vi "Dec.vi"(8 "error in (no error)":errorcluster) -> (0 "error out":errorcluster, 3 "function return":dbl)   [LabVIEW 2014, in "MASTTCSGET.lvlib"]
doc: "gives teliscope declination\n\n\n\n\n__declspec (dllexport) float Dec();"
uses:
  MASTTCSGET.lvlib
  MASTTCSGET.dll
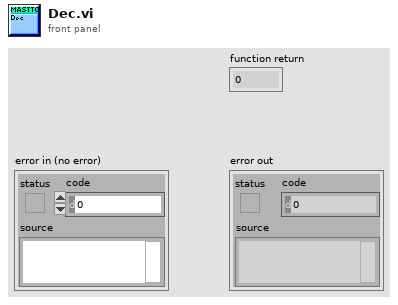
[diagram p1: front panel]
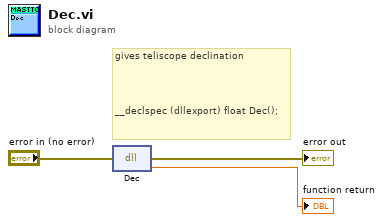
[diagram p0: block diagram]
diagram:
  # "gives teliscope declination\n\n\n\n\n__declspec (dllexport) float Dec();"
  n1 = dll-call lib="F:/weekend/mast_controlsystem/MASTTCSGET.*" fn="Dec"(error in="error in (no error)") -> (error out=→"error out":errorcluster, →"function return":dbl)  [unwired: 2 in, 1 out]
